vi "Delete Dot-Double first end.vi"(11 "String":string) -> (3 "string":string)   [LabVIEW 2021]
panel:
  out "unsigned byte array":u8[](array[numeric])
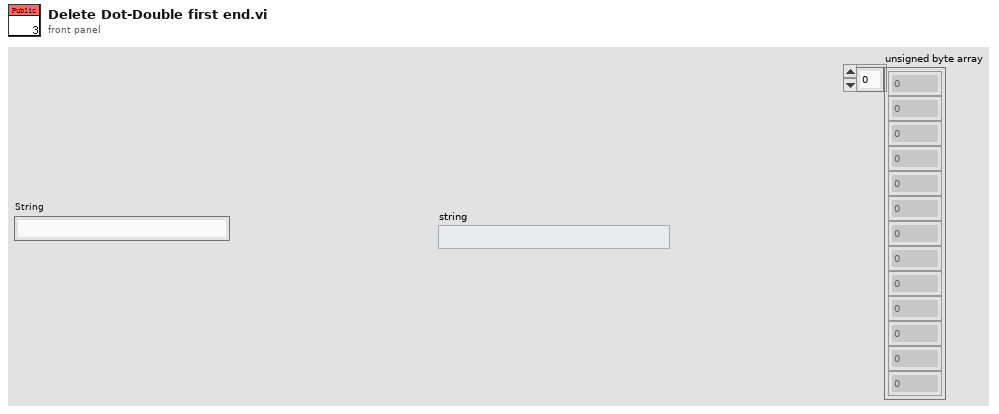
[diagram p1: front panel]
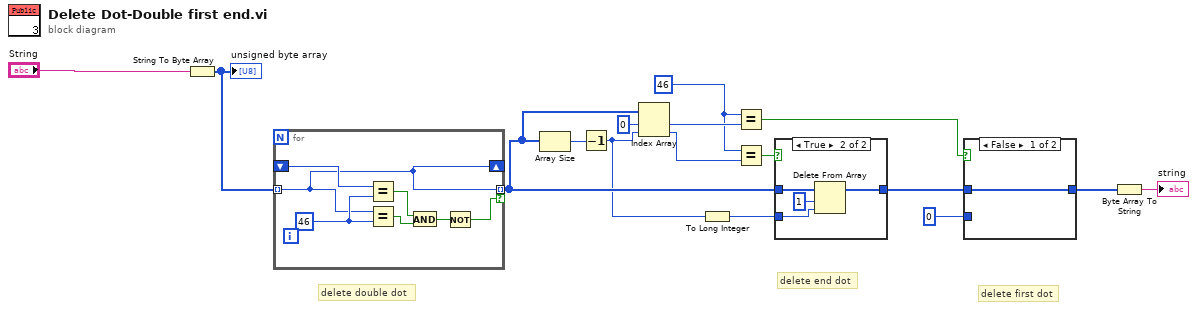
[diagram p0: block diagram]
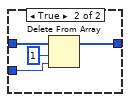
[diagram p2: hidden frame]
diagram:
  w10 = u8 46 ("y")
  # "delete first dot"
  # "delete end dot"
  # "delete double dot"
  n1 = String To Byte Array(string="String") -> (unsigned byte array=w15:u8[])
  "unsigned byte array" <- w15
  n2 = for {
    tunnel: w15 -> [w21] mode=indexing
    shift-right: [w21] -> _
    shift-left: _ -> [w23]
    tunnel: [w21] -> w3 mode=indexing if=w17
    w22 = u8 46 ("y")
    n3 = Equal?(x=w23, y=w22) -> (x = y?=w20:bool)
    n4 = Equal?(x=w21, y=w22) -> (x = y?=w19:bool)
    n5 = And(x=w20, y=w19) -> (x .and. y?=w18:bool)
    n6 = Not(x=w18) -> (.not. x?=w17:bool)
  }
  n7 = Array Size(array=w3) -> (size(s)=w16:i32)
  n8 = Decrement(x=w16) -> (x-1=w1:i32)
  n9 = Index Array(array=w3, index #1=0 ("index"), index #2=w1) -> (element #1=w11:u8, element #2=w9:u8)
  n10 = To Long Integer(number=w1) -> (32bit integer=w7:i32)
  n11 = Equal?(x=w10, y=w11) -> (x = y?=w4:bool)
  n12 = Equal?(x=w10, y=w9) -> (x = y?=w8:bool)
  n13 = case shown="True" w8 {
    tunnel: w3 -> [w24 w28]
    tunnel: w7 -> [_ w26]
    tunnel: [w24 w25] -> w6
    frame False {
    }
    frame True {
      n14 = Delete From Array(array=w28, length=1, index=w26) -> (array with subset deleted=w25:u8[])  [unwired: 1 out]
    }
  }
  n15 = case shown="False" w4 {
    tunnel: w6 -> [w29 w33]
    tunnel: 0 -> [_ w31]
    tunnel: [w29 w30] -> w2
    frame False {
    }
    frame True {
      n16 = Delete From Array(array=w33, length=1, index=w31) -> (array with subset deleted=w30:u8[])  [unwired: 1 out]
    }
  }
  n17 = Byte Array To String(unsigned byte array=w2) -> (string=→"string":string)
